vi "Drive Towards Defender.vi"(4 "defencer angle":dbl, 5 "max forward velocity (m/s)":dbl, 6 "find":bool, 7 "max angular velocity (rad/s)":dbl=1.0, 8 "error in (no error)":errorcluster, 9 "attacker":dbl[](array[numeric]), 10 "defender":dbl[](array[numeric]), 11 "gap":T1) -> (0 "error out":errorcluster, 2 "steering frame velocity":dbl[](array[numeric]))   [LabVIEW 2012]
doc: "Sets the steering frame velocity so that the robot moves towards the gap."
uses:
  <vilib>/robotics/Obstacle Avoidance/Simple Vector Field Histogram/Gap Description.ctl
  <vilib>/imath/engines/lvmath2/RunTimeEngine/NodeEndStatement/NIMS_NodeEndStatement_Output.vi
  <instcachedir>/0/NIMS_NodeEndStatement_Output_53EC0D466D134D7ABD903AC30B43404B.lvgen/NIMS_NodeEndStatement_Output_53EC0D466D134D7ABD903AC30B43404B_001.vi
  <vilib>/imath/engines/lvmath2/RunTimeEngine/BuiltInFunctions/atan2/NIMS_atan2.vi
  <instcachedir>/0/NIMS_atan2_A91AA4A7D42247EDBE8F76DB99AF04A4.lvgen/NIMS_atan2_A91AA4A7D42247EDBE8F76DB99AF04A4_001.vi
  <vilib>/imath/engines/lvmath2/RunTimeEngine/ErrorHandling/NIMS_Finalize Error.vi
  <vilib>/robotics/Obstacle Avoidance/Simple Vector Field Histogram/NI_Robotics_Simple Vector Field Histogram.lvlib
panel:
  out "find 2":bool
  out "angle 3":dbl
  out "angle 2":dbl(knob) scale=-1.2..1.2
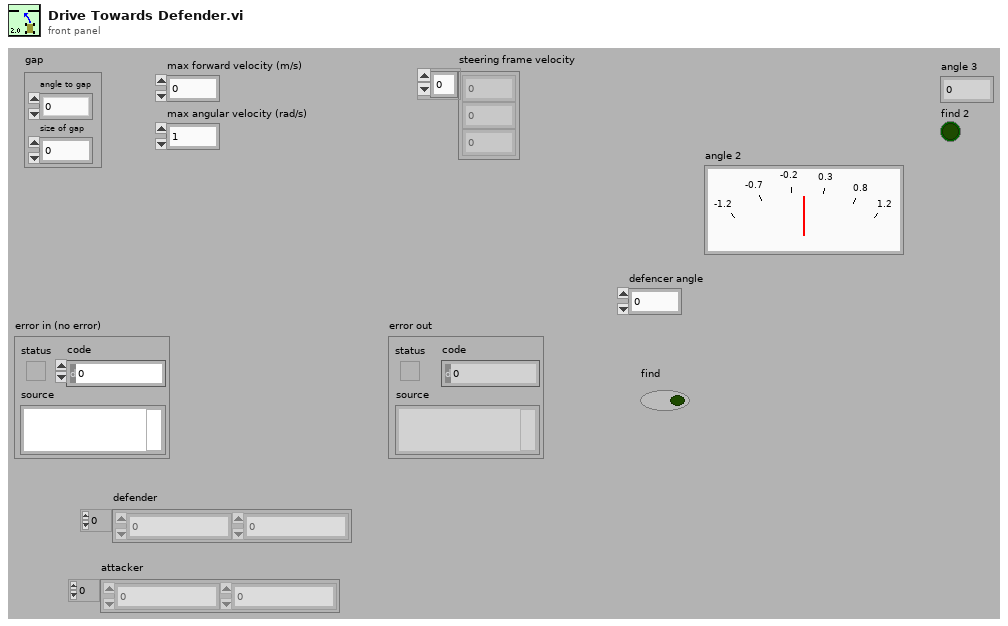
[diagram p1: front panel]
types:
  T1 = typedef "NI_Robotics_Simple Vector Field Histogram.lvlib/Gap Description.ctl" = cluster{"angle to gap":dbl, "size of gap":dbl}
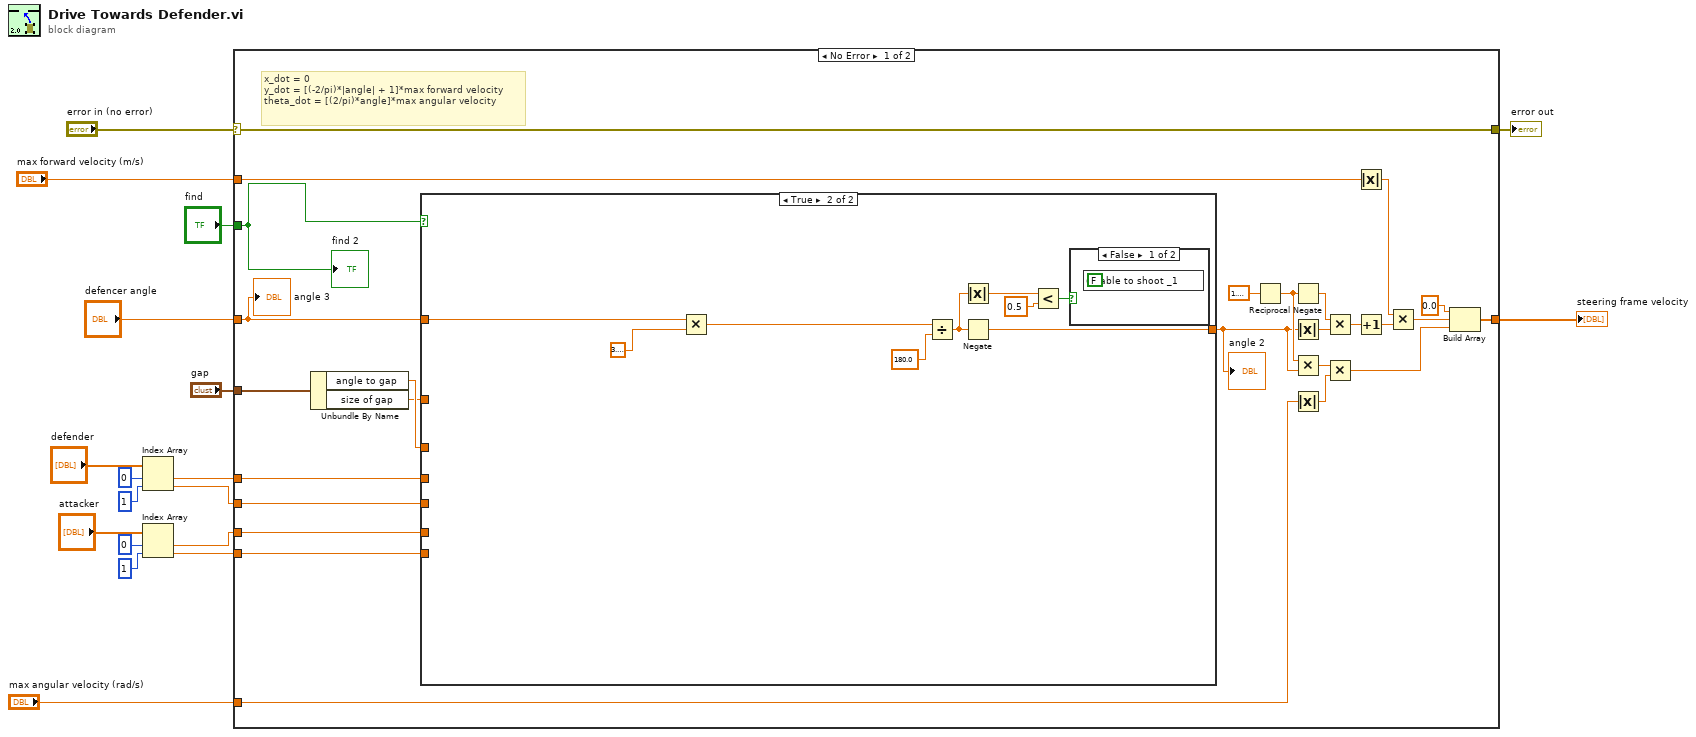
[diagram p0: block diagram]
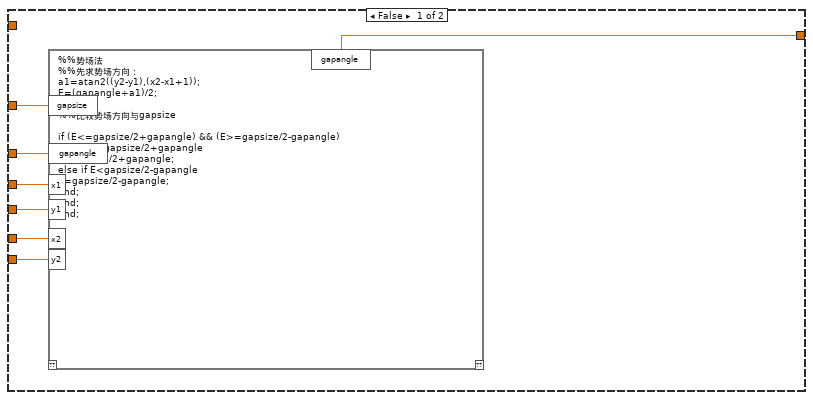
[diagram p2: hidden frame]
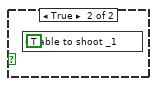
[diagram p3: hidden frame]
diagram:
  n1 = Index Array(array="defender", index #1=0 ("index"), index #2=1 ("index")) -> (element #1=w6:dbl, element #2=w5:dbl)
  n2 = Index Array(array="attacker", index #1=0 ("index"), index #2=1 ("index")) -> (element #1=w4:dbl, element #2=w3:dbl)
  n3 = case shown="No Error" "error in (no error)" {
    selector: "error in (no error)" -> [w43 w144]
    tunnel: "gap" -> [w44 _]
    tunnel: [w43 w144] -> w16
    tunnel: "max forward velocity (m/s)" -> [w38 _]
    tunnel: "max angular velocity (rad/s)" -> [w35 _]
    tunnel: [w31 _] -> w13
    tunnel: w6 -> [w25 _]
    tunnel: w5 -> [w24 _]
    tunnel: w4 -> [w23 _]
    tunnel: w3 -> [w22 _]
    tunnel: "defencer angle" -> [w20 _]
    tunnel: "find" -> [w19 _]
    frame No Error {
      # "x_dot = 0\ny_dot = [(-2/pi)*|angle| + 1]*max forward velocity\ntheta_dot = [(2/pi)*angle]*max angular velocity"
      n4 = Unbundle By Name(w44) -> ("angle to gap"=w27:dbl, "size of gap"=w21:dbl)
      n5 = case shown="True" w19 {
        tunnel: w27 -> [w51 _]
        tunnel: [w45 w138] -> w26
        tunnel: w25 -> [w50 _]
        tunnel: w24 -> [w49 _]
        tunnel: w23 -> [w48 _]
        tunnel: w22 -> [w47 _]
        tunnel: w21 -> [w46 _]
        tunnel: w20 -> [_ w135]
        frame False {
          n6 = mathscript code="%%势场法\n%%先求势场方向：\na1=atan2((y2-y1),(x2-x1+1));\nE=(gapangle+a1)/2;\n\n%%比较势场方向与gapsize\n\nif (E<=gapsize/2+gapangle) && (E>=gapsize/2-gapangle)\nelse if E>gapsize/2+gapangle\nE=gapsize/2+gapangle;\nelse if E<gapsize/2-gapangle\nE=gapsize/2-gapangle;\nend;\nend;\nend;"("gapangle"=w51, "x1"=w50, "y1"=w49, "x2"=w48, "y2"=w47, "gapsize"=w46) -> ("gapangle"=w45:dbl)  [unwired: 1 in, 1 out]
        }
        frame True {
          n7 = Multiply(x=w135, y=3.141592653589793) -> (x*y=w136:dbl)
          n8 = Divide(x=w136, y=180.0) -> (x/y=w137:dbl)
          n9 = Absolute Value(x=w137) -> (abs(x)=w139:dbl)
          n10 = Negate(x=w137) -> (-x=w138:dbl)
          n11 = Less?(x=w139, y=0.5) -> (x < y?=w141:bool)
          n12 = case shown="False" w141 {
            frame False {
              n13 = global write "Global of computer.vi" "able to shoot _1"(FALSE ("shoot")) -> ()
            }
            frame True {
              n14 = global write "Global of computer.vi" "able to shoot _1"(TRUE ("shoot")) -> ()
            }
          }
        }
      }
      "angle 2" <- w26
      n15 = Reciprocal(x=1.5707963267948966) -> (1/x=w37:dbl)
      n16 = Negate(x=w37) -> (-x=w41:dbl)
      n17 = Absolute Value(x=w26) -> (abs(x)=w28:dbl)
      n18 = Multiply(x=w37, y=w26) -> (x*y=w36:dbl)
      n19 = Absolute Value(x=w35) -> (abs(x)=w29:dbl)
      n20 = Multiply(x=w41, y=w28) -> (x*y=w40:dbl)
      n21 = Multiply(x=w36, y=w29) -> (x*y=w33:dbl)
      n22 = Absolute Value(x=w38) -> (abs(x)=w30:dbl)
      n23 = Increment(x=w40) -> (x+1=w39:dbl)
      n24 = Multiply(x=w30, y=w39) -> (x*y=w34:dbl)
      n25 = Build Array(0.0 ("element"), w34, w33) -> (w31:dbl[])
      "angle 3" <- w20
      "find 2" <- w19
    }
    frame Error {
    }
  }
  "error out" <- w16
  "steering frame velocity" <- w13
